vi "time srting.vi"() -> (3 "date/time string":string)   [LabVIEW 2016]
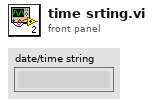
[diagram p1: front panel]
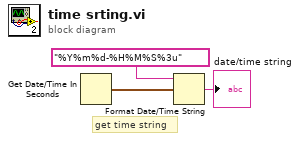
[diagram p0: block diagram]
diagram:
  # "get time string"
  n1 = Get Date/Time In Seconds() -> (seconds since 1Jan1904=w2:timestamp)
  n2 = Format Date/Time String(time format string (%c)="%Y%m%d-%H%M%S%3u", seconds (now)=w2) -> (date/time string=→"date/time string":string)  [unwired: 1 in]
